vi "Initialize.vi"(8 "error in":errorcluster, 10 "shared resources":refnum<class "Shared Resources.lvclass">, 11 "Tx Execution Unit Implementation in":refnum<class "Tx Execution Unit.lvclass">) -> (0 "error out":errorcluster, 3 "Tx Execution Unit Implementation out":refnum<class "Tx Execution Unit.lvclass">)   [LabVIEW 2020, in "Ballard MIL-STD-1553 Engine.lvlib" / "Implementation.lvlib" / "Tx Execution Unit.lvclass"]
uses:
  Tx Execution Unit.lvclass
  Execution Unit/Execution Unit.lvclass
  Custom Device/Custom Device.lvlib
  C:/Users/nitest/Desktop/Git 2020/niveristand-aim-milStd1553-custom-device/Source/Custom Device Support/Engine/Implementation/Execution Unit/Execution Unit.lvclass
  C:/Users/nitest/Desktop/Git 2020/niveristand-aim-milStd1553-custom-device/Source/Custom Device Support/Engine/Interfaces/Execution Unit/Execution Unit.lvclass
  C:/Users/nitest/Desktop/Git 2020/niveristand-aim-milStd1553-custom-device/Source/Custom Device Support/Engine/Implementation/Tx Execution Unit/Tx Execution Unit.lvclass
  Interfaces/Shared Resources/Shared Resources.lvclass
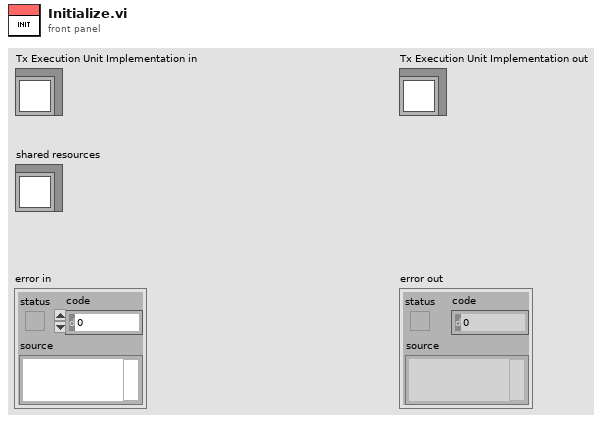
[diagram p1: front panel]
types:
  T1 = typedef "1553 Channel.ctl" = cluster{"HW channel":u16, "terminal addresses":T2[], "terminal names":string[], "acyclic frame names":string[], "messages":T3[]}
  T2 = typedef "Address.ctl" = u16
  T3 = typedef "Message Definition.ctl" = cluster{"name":string, "message type":T4, "endpoint Tx":T5, "endpoint Rx":T5, "create timestamp channel":bool, "mode code":u16, "number of words":u16, "parameters":cluster{"name":string, "default value":dbl, "unit":string, "parameter definition":T6}[]}
  T4 = typedef "Message Type.ctl" = string
  T5 = typedef "Terminal Endpoint.ctl" = cluster{"terminal address":T2, "subaddress":T2}
  T6 = typedef "Parameter Definition.ctl" = cluster{"start index":i32, "size (bits)":i32, "encoding":enum16{"BNR", "BCD", "Discrete"}, "signed":bool, "multiplier":dbl, "offset":dbl}
  T7 = typedef "Ballard MIL-STD-1553 Engine.lvlib/Custom Device.lvlib/Hardware Handles.ctl" = cluster{"core handle":u64, "core reader handle":u64, "channel handles":u64[]}
  T8 = typedef "Ballard MIL-STD-1553 Engine.lvlib/Implementation.lvlib/Execution Unit.lvclass/1553 Channel Handles.ctl" = cluster{"messages":T9[], "error count channel refs":T12, "terminal status channels":T11[]}
  T9 = typedef "Ballard MIL-STD-1553 Engine.lvlib/Implementation.lvlib/Execution Unit.lvclass/Message Handles.ctl" = cluster{"parameters":T10[], "timestamps":T11[], "Tx status handles":T11[], "Rx status handles":T11[]}
  T10 = typedef "Ballard MIL-STD-1553 Engine.lvlib/Implementation.lvlib/Execution Unit.lvclass/Parameter Handles.ctl" = cluster{"Tx channel handle":T11, "RxRT channel handle":T11, "RxBC channel handle":T11}
  T11 = typedef "Custom Device API.lvlib/Custom Device Item Ref.ctl" = u64
  T12 = typedef "Error Count Channel Refs.ctl" = cluster{"general protocol":T11, "improper number of words":T11, "Manchester":T11, "monitor":T11, "parity":T11, "unconfigured frames":T11, "word":T11, "wrong sync":T11}
  T13 = typedef "Map of Message Indexes to Tx Write Info.ctl" = map{i32, T14}
  T14 = typedef "Tx Write Info.ctl" = cluster{"transfer handle":u64, "value index":i32}
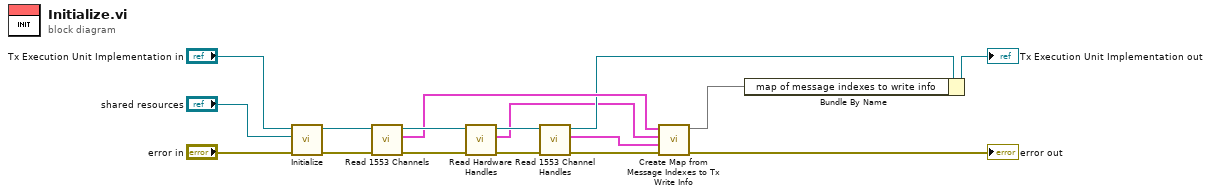
[diagram p0: block diagram]
diagram:
  n1 = call-parent "Initialize.vi"("error in"="error in", "shared resources"="shared resources", "Execution Unit Implementation in"="Tx Execution Unit Implementation in") -> ("error out"=w12:errorcluster, "Execution Unit Implementation out"=w14:refnum<class "Tx Execution Unit.lvclass">)  [unwired: 7 in]
  n2 = call "Read 1553 Channels.vi"("error in"=w12, "Execution Unit in"=w14) -> ("error out"=w10:errorcluster, "1553 channels"=w8:T1[], "Execution Unit out"=w9:refnum<class "Tx Execution Unit.lvclass">)  [unwired: 7 in]
  n3 = call "Read Hardware Handles.vi"("error in"=w10, "Execution Unit in"=w9) -> ("error out"=w4:errorcluster, "hardware handles"=w1:T7, "Execution Unit out"=w6:refnum<class "Tx Execution Unit.lvclass">)  [unwired: 7 in]
  n4 = call "Read 1553 Channel Handles.vi"("error in"=w4, "Execution Unit in"=w6) -> ("error out"=w3:errorcluster, "1553 channel handles"=w2:T8[], "Execution Unit out"=w5:refnum<class "Tx Execution Unit.lvclass">)  [unwired: 7 in]
  n5 = call "Create Map from Message Indexes to Tx Write Info.vi"("error in"=w3, "1553 channel handles"=w2, "hardware handles"=w1, "1553 channels"=w8) -> ("error out"=→"error out":errorcluster, "map from message indexes to Tx write info"=w7:T13)  [unwired: 6 in]
  n6 = Bundle By Name(cluster=w5, "map of message indexes to write info"=w7) -> (→"Tx Execution Unit Implementation out":refnum<class "Tx Execution Unit.lvclass">)
